vi "SetDisplayState.vi"(8 "Error In":errorcluster, 10 "Enabled?":bool, 11 "Keithley 6482 In":refnum<visa-resource-name>) -> (0 "Error Out":errorcluster, 3 "Keithley 6482 Out":refnum<visa-resource-name>)   [LabVIEW 8.6, in "Keithley-6482-Visa.lvlib"]
uses:
  Keithley-6482-Visa.lvlib
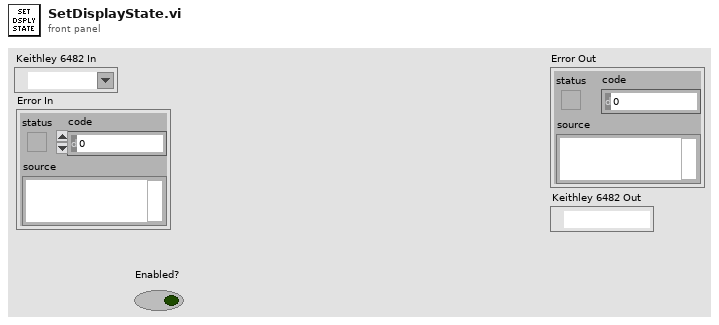
[diagram p1: front panel]
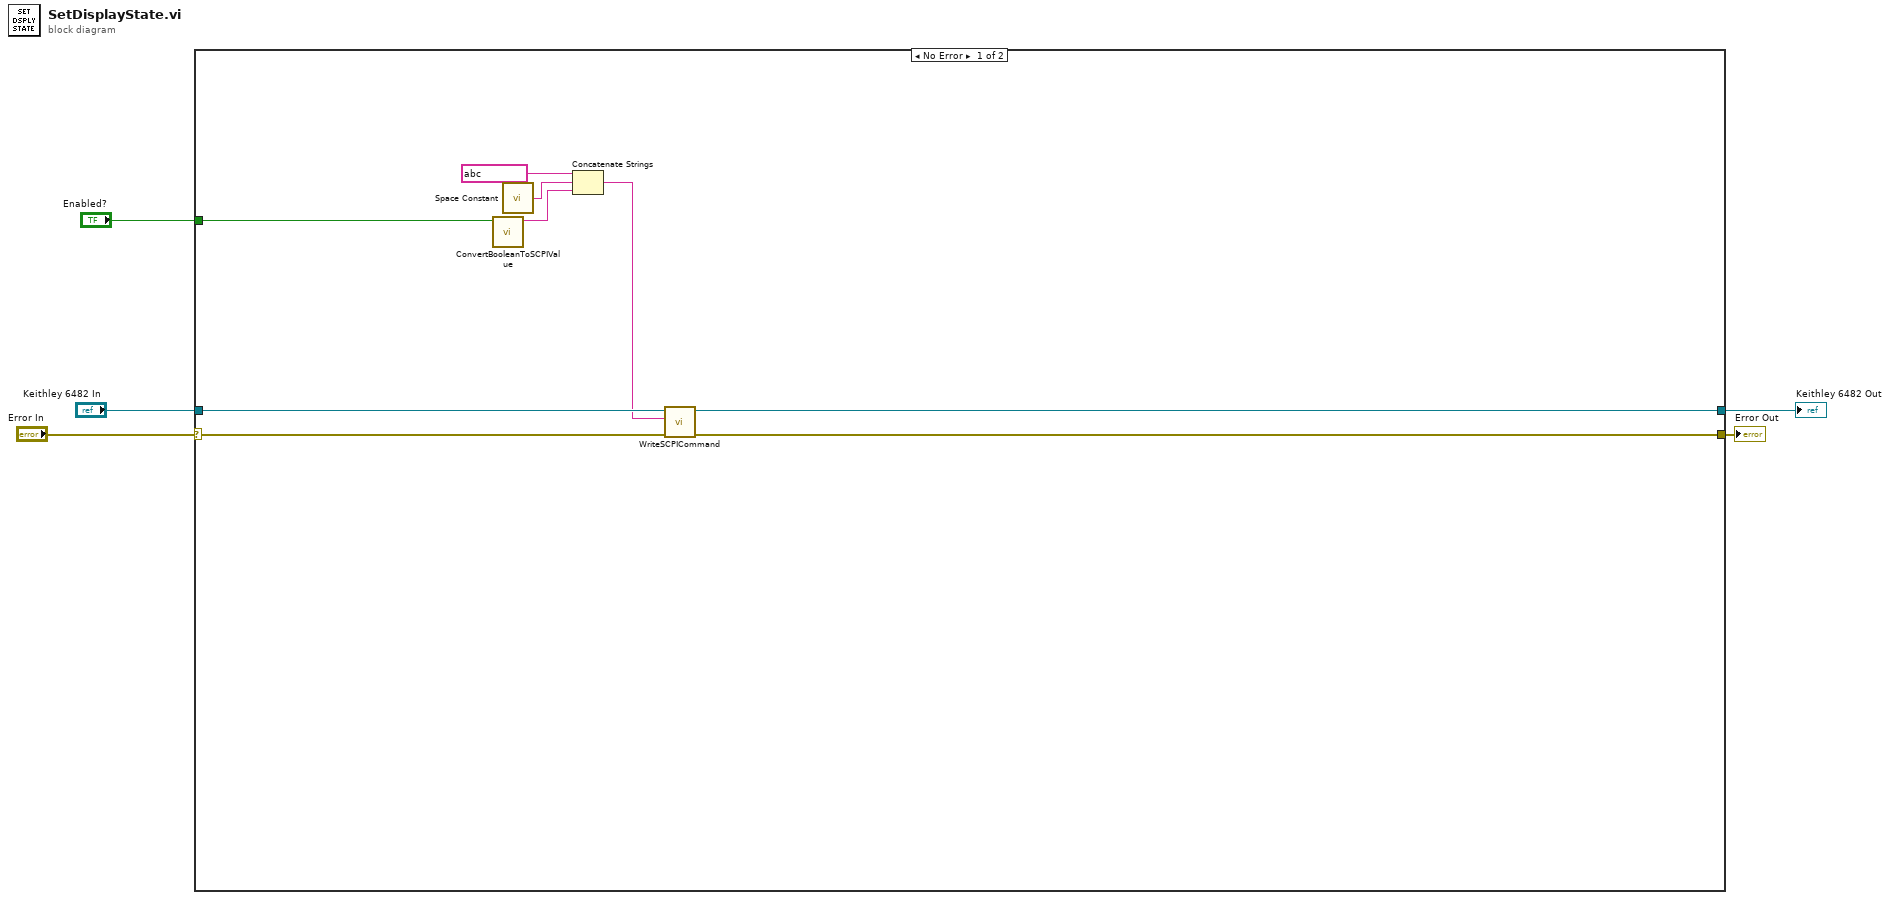
[diagram p0: block diagram]
diagram:
  n1 = case shown="No Error" "Error In" {
    selector: "Error In" -> [w7 w15]
    tunnel: "Keithley 6482 In" -> [w10 w16]
    tunnel: [w8 w15] -> w3
    tunnel: [w9 w16] -> w2
    tunnel: "Enabled?" -> [w14 _]
    frame #0 {
      n2 = call "ConvertBooleanToSCPIValue.vi"("Boolean"=w14) -> ("SCPI Value"=w11:string)  [unwired: 10 in]
      n3 = call <vilib>:"Space Constant.vi"() -> ("String"=w12:string)
      n4 = Concatenate Strings(string ?, w12, w11) -> (w6:string)
      n5 = call "WriteSCPICommand.vi"("Error In"=w7, "SCPI Command"=w6, "Keithley 6482 In"=w10) -> ("Error Out"=w8:errorcluster, "Keithley 6482 Out"=w9:refnum<visa-resource-name>)  [unwired: 7 in]
    }
    frame #1 {
    }
  }
  "Error Out" <- w3
  "Keithley 6482 Out" <- w2
